vi "Check Syntax.vi"(8 "error in (no error)":errorcluster, 10 "Segments in":T2[](array[typedef]), 11 "ProtoParser in":refnum<class "ProtoParser.lvclass">) -> (0 "error out":errorcluster, 2 "Segments":T2[](array[typedef]), 3 "ProtoParser out":refnum<class "ProtoParser.lvclass">, 5 "Syntax":T1)   [LabVIEW 2020, in "LV-Protoc.lvlib" / "ProtoParser.lvclass"]
uses:
  ProtoParser.lvclass
  Raw Segment.ctl
  Segment Type.ctl
  Syntax.ctl
  LV-Protoc.lvlib
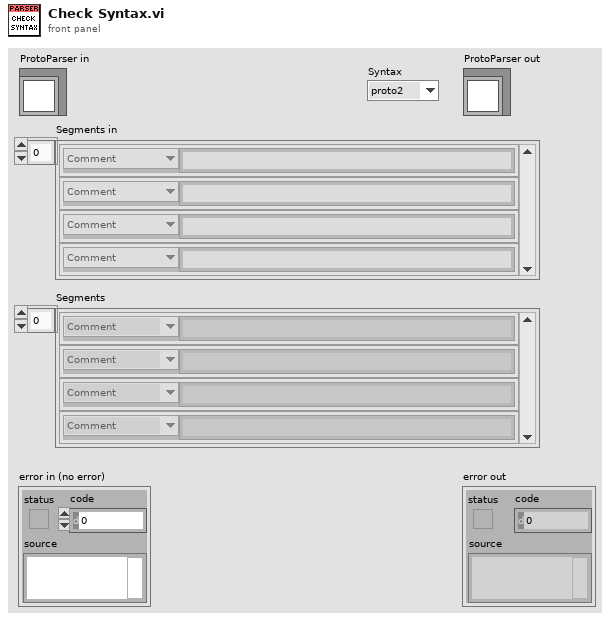
[diagram p1: front panel]
types:
  T1 = typedef "LV-Protoc.lvlib/Syntax.ctl" = enum16{"proto2", "proto3"}
  T2 = typedef "LV-Protoc.lvlib/Raw Segment.ctl" = cluster{"Type":T3, "Text":string}
  T3 = typedef "LV-Protoc.lvlib/Segment Type.ctl" = enum16{"Comment", "Message Open", "Enum Open", "Message Close", "Enum Close", "Field", "Syntax", "Import", "Enum Value", "Package", "Reserved"}
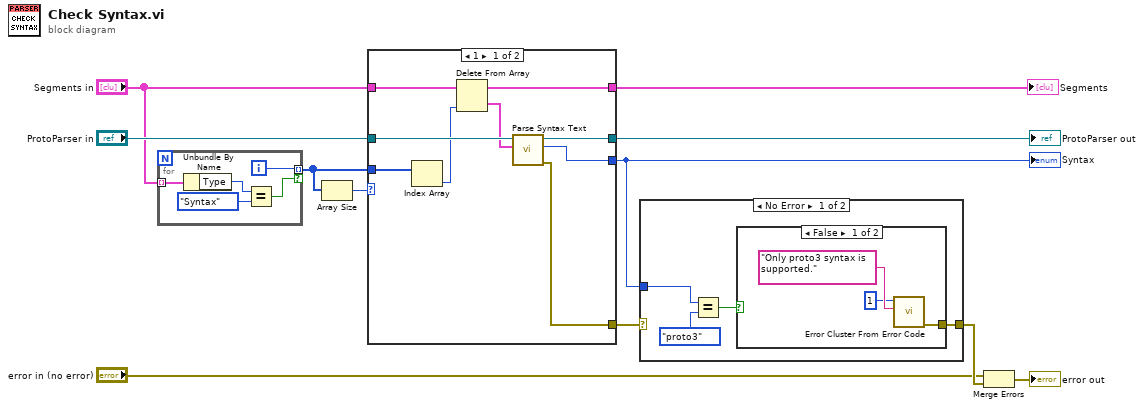
[diagram p0: block diagram]
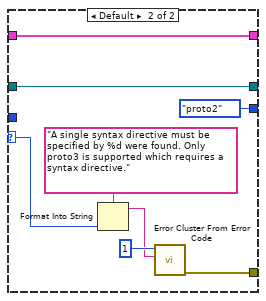
[diagram p2: hidden frame]
diagram:
  n1 = for {
    tunnel: "Segments in" -> [w16] mode=indexing
    tunnel: [w13] -> w2 mode=indexing if=w12
    i -> [w13]
    n2 = Unbundle By Name(w16) -> ("Type"=w15:T3)
    n3 = Equal?(x=w15, y=Segment_Type."Syntax") -> (x = y?=w12:bool)
  }
  n4 = Array Size(array=w2) -> (size(s)=w11:i32)
  n5 = case shown="1" w11 {
    selector: w11 -> [_ w30]
    tunnel: "ProtoParser in" -> [w25 w33]
    tunnel: [w24 w33] -> w9
    tunnel: [w23 w28] -> w8
    tunnel: [w22 Syntax."proto2" ("Syntax")] -> w7
    tunnel: "Segments in" -> [w20 w26]
    tunnel: w2 -> [w21 _]
    tunnel: [w17 w26] -> w1
    frame 1 {
      n6 = Index Array(array=w21) -> (element=w19:i32)  [unwired: 1 in]
      n7 = Delete From Array(array=w20, index=w19) -> (deleted portion=w18:T2, array with subset deleted=w17:T2[])  [unwired: 1 in]
      n8 = call "Parse Syntax Text.vi"("Segment"=w18, "ProtoParser in"=w25) -> ("error out"=w23:errorcluster, "Syntax"=w22:T1, "ProtoParser out"=w24:refnum<class "ProtoParser.lvclass">)  [unwired: 7 in]
    }
    frame Default {
      n9 = Format Into String(format string="A single syntax directive must be specified by %d were found. Only proto3 is supported which requires a syntax directive.", w30) -> (resulting string=w29:string)  [unwired: 2 in, 1 out]
      n10 = call <vilib>:"Error Cluster From Error Code.vi"("error message (\"\")"=w29, "error code (0)"=1) -> ("error out"=w28:errorcluster)  [unwired: 7 in]
    }
  }
  "ProtoParser out" <- w9
  "Segments" <- w1
  "Syntax" <- w7
  n11 = case shown="No Error" w8 {
    selector: w8 -> [_ w41]
    tunnel: w7 -> [w35 _]
    tunnel: [w34 w41] -> w6
    frame No Error {
      n12 = Equal?(x=w35, y=Syntax."proto3" ("Syntax")) -> (x = y?=w36:bool)
      n13 = case shown="False" w36 {
        tunnel: [w40 _] -> w34
        frame False {
          n14 = call <vilib>:"Error Cluster From Error Code.vi"("error message (\"\")"="Only proto3 syntax is supported.", "error code (0)"=1) -> ("error out"=w40:errorcluster)  [unwired: 7 in]
        }
        frame True {
        }
      }
    }
    frame Error {
    }
  }
  n15 = Merge Errors("error in (no error)", w6) -> (→"error out":errorcluster)
